vi "h.ACQ.ParseGetSpectrumHeader.vi"(11 "Header from #GetSpectrum":u8[](array[numeric])) -> (0 "Channels":u16, 1 "Time Stamp (ns)":u64, 2 "SN":u64, 3 "Header Length":u16, 4 "Wvl Inc":dbl, 5 "Num Points":u32, 6 "Start Wvl":dbl)   [LabVIEW 2019, in "h.Library.lvlib"]
doc: "This vi parses the header returned by the #GetSpectrum command and returns the contained data through a number of outputs.\n\n<b>Header from #GetSpectrum</b> - data returned by h.DAQ.GetSpectrum.vi\n<b>Header Length</b> - The total header length in bytes (also the start of the peaks data)s\n<b>SN</b> - Serial Number of the collected data set\n<b>Time Stamp</b> - The estimated time in ns when the instrument acquired the spectrum\n<b>Start Wvl</b> - Wvl of the first data point in nm\n<b>Wvl Inc</b> - Wavelength increment between sample points in nm\n<b>NumSpectra</b> - The number of spectra transfered\n<b>Num Points</b> - The number of data points in each transfered spectrum"
uses:
  h.Library.lvlib
panel:
  out "Reserved 2":u16
  out "Reserved":u32
  out "Header Version":u16
  # "Hyperion Parse #GetSpectrum Header"
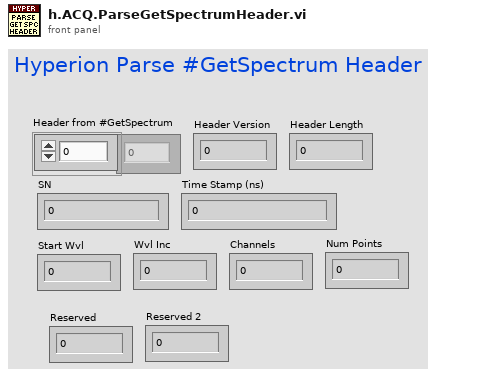
[diagram p1: front panel]
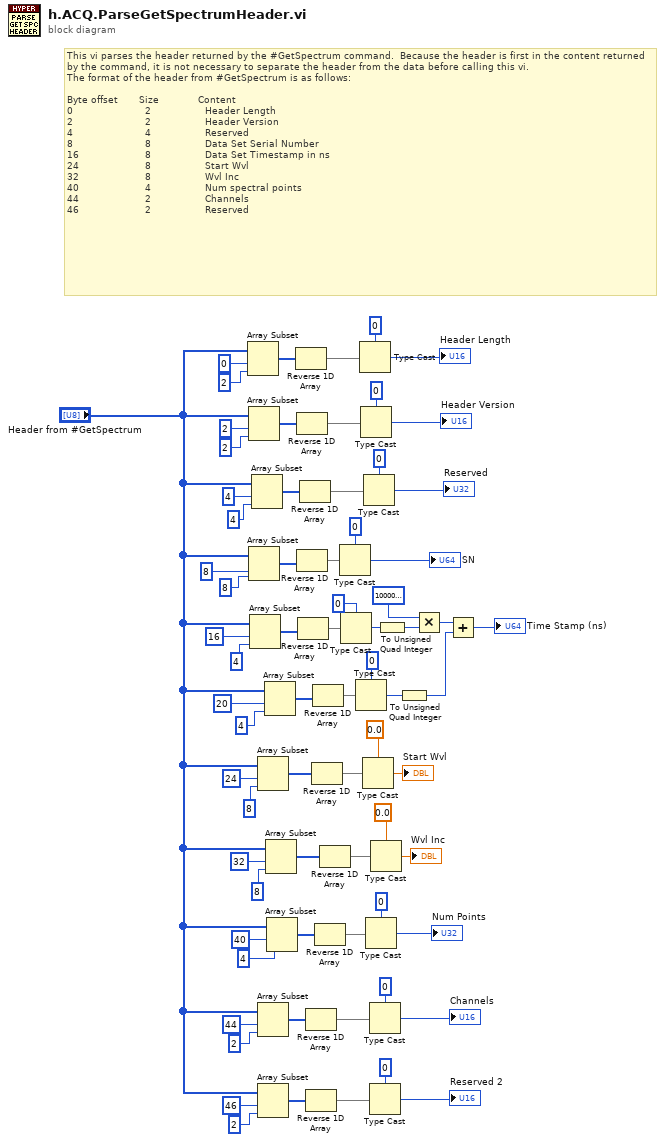
[diagram p0: block diagram]
diagram:
  # "This vi parses the header returned by the #GetSpectrum command.  Because the header is first in the content returned by the command, it is not necessary to separate the header from the data before calling this vi.\nThe format of the header from #GetSpectrum is as follows:\n\nByte offset       Size             Content\n0                        2                  Header Length\n2                        2                  Header Version\n4                        4                  Reserved\n8                        8                  Data Set Serial Number\n16                      8                  Data Set Timestamp in ns\n24                      8                  Start Wvl\n32                      8                  Wvl Inc\n40                      4                  Num spectral points\n44                      2                  Channels\n46                      2                  Reserved"
  n1 = Array Subset(array="Header from #GetSpectrum", index=0, length=2) -> (w38:u8[])
  n2 = Array Subset(array="Header from #GetSpectrum", index=2, length=2) -> (w63:u8[])
  n3 = Array Subset(array="Header from #GetSpectrum", index=8, length=8) -> (w50:u8[])
  n4 = Array Subset(array="Header from #GetSpectrum", index=16, length=4) -> (w44:u8[])
  n5 = Array Subset(array="Header from #GetSpectrum", index=4, length=4) -> (w17:u8[])
  n6 = Array Subset(array="Header from #GetSpectrum", index=24, length=8 ("y")) -> (w35:u8[])
  n7 = Array Subset(array="Header from #GetSpectrum", index=44, length=2) -> (w11:u8[])
  n8 = Array Subset(array="Header from #GetSpectrum", index=46, length=2) -> (w4:u8[])
  n9 = Array Subset(array="Header from #GetSpectrum", index=20, length=4) -> (w66:u8[])
  n10 = Array Subset(array="Header from #GetSpectrum", index=32, length=8 ("y")) -> (w29:u8[])
  n11 = Array Subset(array="Header from #GetSpectrum", index=40, length=4) -> (w22:u8[])
  n12 = Reverse 1D Array(array=w38) -> (reversed array=w39:u8[])
  n13 = Reverse 1D Array(array=w63) -> (reversed array=w64:u8[])
  n14 = Reverse 1D Array(array=w50) -> (reversed array=w49:u8[])
  n15 = Reverse 1D Array(array=w44) -> (reversed array=w46:u8[])
  n16 = Reverse 1D Array(array=w17) -> (reversed array=w18:u8[])
  n17 = Reverse 1D Array(array=w11) -> (reversed array=w12:u8[])
  n18 = Reverse 1D Array(array=w4) -> (reversed array=w5:u8[])
  n19 = Reverse 1D Array(array=w35) -> (reversed array=w34:u8[])
  n20 = Reverse 1D Array(array=w66) -> (reversed array=w56:u8[])
  n21 = Reverse 1D Array(array=w22) -> (reversed array=w23:u8[])
  n22 = Reverse 1D Array(array=w29) -> (reversed array=w28:u8[])
  n23 = Type Cast(type=u64 0 ("length"), x=w49) -> (*(type *) &x=→"SN":u64)
  n24 = Type Cast(type=u32 0 ("length"), x=w46) -> (*(type *) &x=w61:u32)
  n25 = Type Cast(type=u32 0 ("length"), x=w56) -> (*(type *) &x=w60:u32)
  n26 = Type Cast(type=u16 0 ("length"), x=w39) -> (*(type *) &x=→"Header Length":u16)
  n27 = Type Cast(type=u16 0 ("length"), x=w64) -> (*(type *) &x=→"Header Version":u16)
  n28 = Type Cast(type=0.0, x=w34) -> (*(type *) &x=→"Start Wvl":dbl)
  n29 = Type Cast(type=u32 0 ("length"), x=w18) -> (*(type *) &x=→"Reserved":u32)
  n30 = Type Cast(type=u32 0 ("length"), x=w23) -> (*(type *) &x=→"Num Points":u32)
  n31 = Type Cast(type=u16 0 ("length"), x=w12) -> (*(type *) &x=→"Channels":u16)
  n32 = Type Cast(type=u16 0 ("length"), x=w5) -> (*(type *) &x=→"Reserved 2":u16)
  n33 = Type Cast(type=0.0, x=w28) -> (*(type *) &x=→"Wvl Inc":dbl)
  n34 = To Unsigned Quad Integer(1:w61) -> (0:w71:u64)
  n35 = To Unsigned Quad Integer(1:w60) -> (0:w59:u64)
  n36 = Multiply(x=u64 1000000000 ("y"), y=w71) -> (x*y=w58:u64)
  n37 = Add(x=w58, y=w59) -> (x+y=→"Time Stamp (ns)":u64)
